vi "Config LAN Trigger.vi"(0 "VISA resource name":refnum<visa-resource-name>, 1 "Mode (Either)":T1(ring), 2 "IP Address":string, 3 "Protocol (TCP)":enum16{"TCP", "UDP", "Multicast"}(ring), 5 "Node In":string, 7 "Trigger # (1)":u32=1 min=1 max=8, 9 "Input Event":string="0", 11 "error in":errorcluster, 12 "Initial Line State (High)":bool=TRUE) -> (4 "VISA resource name out":refnum<visa-resource-name>, 6 "Node Out":string, 14 "Command String":string, 15 "error out":errorcluster)   [LabVIEW 2018, in "Keithley 2600 Series.lvlib"]
doc: "This VI configures a LAN trigger in the advanced trigger model.\n\nThis VI does not connect the LAN trigger. Call LAN Trigger Connect.vi after calling this VI to connect.\n\n<b>Functions and Attributes Used</b>\nlan.trigger[n].ipaddress\nlan.trigger[n].mode\nlan.trigger[n].protocol\nlan.trigger[n].pseudostate\nlan.trigger[n].stimulus"
uses:
  Keithley 2600 Series.lvlib
  Private/GlobalVariables.vi
panel:
  # "(c) 2008 Keithley Instruments, Inc.  ALL RIGHTS RESERVED."
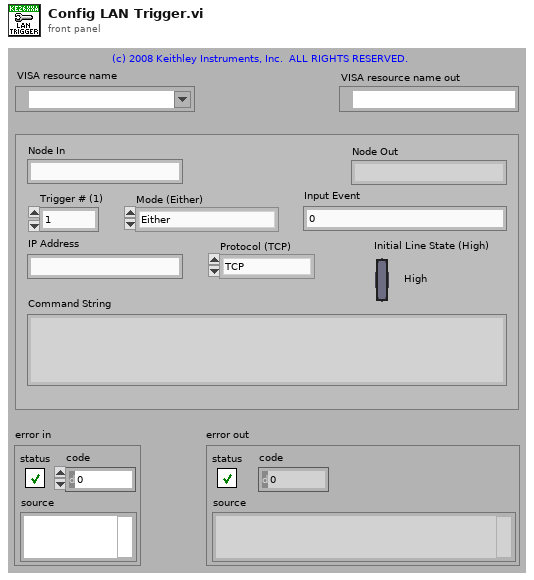
[diagram p1: front panel]
types:
  T1 = enum16{"Either", "Falling", "Rising", "Rising Acceptor", "Rising Master", "Synchronous", "Synchronous Acceptor", "Syncronous Master"}
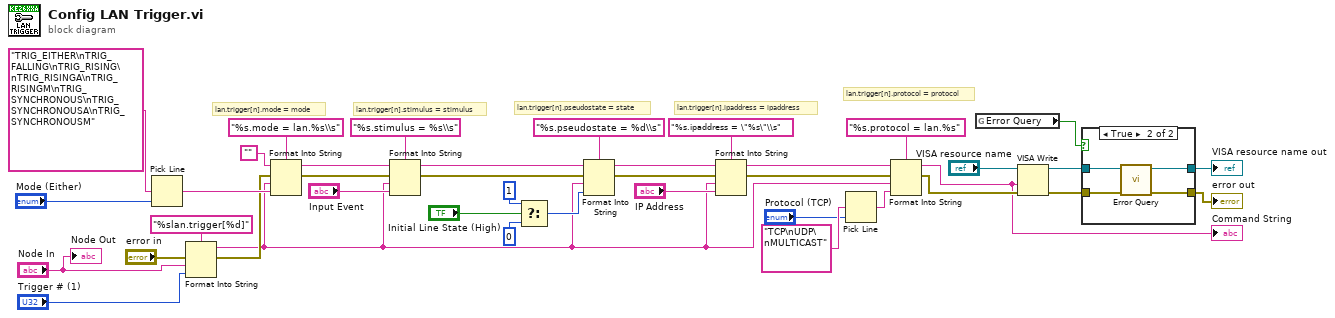
[diagram p0: block diagram]
diagram:
  # "lan.trigger[n].protocol = protocol"
  # "lan.trigger[n].ipaddress = ipaddress"
  # "lan.trigger[n].pseudostate = state"
  # "lan.trigger[n].stimulus = stimulus"
  # "lan.trigger[n].mode = mode"
  n1 = Pick Line(multi-line string="TRIG_EITHER\nTRIG_FALLING\nTRIG_RISING\nTRIG_RISINGA\nTRIG_RISINGM\nTRIG_SYNCHRONOUS\nTRIG_SYNCHRONOUSA\nTRIG_SYNCHRONOUSM", line index="Mode (Either)") -> (output string=w22:string)  [unwired: 1 out]
  n2 = Format Into String(format string="%slan.trigger[%d]", error in="error in", "Node In", "Trigger # (1)") -> (resulting string=w9:string, error out=w21:errorcluster)  [unwired: 1 in]
  n3 = Format Into String(format string="%s.mode = lan.%s\\s", initial string="", error in=w21, w9, w22) -> (resulting string=w35:string, error out=w36:errorcluster)
  n4 = Format Into String(format string="%s.stimulus = %s\\s", initial string=w35, error in=w36, w9, "Input Event") -> (resulting string=w28:string, error out=w29:errorcluster)
  n5 = Select(t=u32 1, s="Initial Line State (High)", f=u32 0) -> (s? t:f=w19:u32)
  n6 = Format Into String(format string="%s.pseudostate = %d\\s", initial string=w28, error in=w29, w9, w19) -> (resulting string=w16:string, error out=w17:errorcluster)
  n7 = Format Into String(format string="%s.ipaddress = \"%s\"\\s", initial string=w16, error in=w17, w9, "IP Address") -> (resulting string=w11:string, error out=w12:errorcluster)
  n8 = Pick Line(multi-line string="TCP\nUDP\nMULTICAST", line index="Protocol (TCP)") -> (output string=w10:string)  [unwired: 1 out]
  n9 = Format Into String(format string="%s.protocol = lan.%s", initial string=w11, error in=w12, w9, w10) -> (resulting string=w1:string, error out=w8:errorcluster)
  "Command String" <- w1
  n10 = global read "GlobalVariables.vi" "Error Query"() -> (w4:bool)
  n11 = VISA Write(VISA resource name="VISA resource name", write buffer=w1, error in (no error)=w8) -> (VISA resource name out=w6:refnum<visa-resource-name>, error out=w5:errorcluster)  [unwired: 1 out]
  n12 = case shown="True" w4 {
    tunnel: w6 -> [w42 w46]
    tunnel: w5 -> [w41 w45]
    tunnel: [w42 w44] -> w3
    tunnel: [w41 w43] -> w2
    frame False {
    }
    frame True {
      n13 = call "Error Query.vi"("error in (no error)"=w45, "VISA resource name"=w46) -> ("error out"=w43:errorcluster, "VISA resource name out"=w44:refnum<visa-resource-name>)  [unwired: 8 out]
    }
  }
  "VISA resource name out" <- w3
  "error out" <- w2
  "Node Out" <- "Node In"
